vi "Global_MAIN.vi"() -> ()   [LabVIEW 2015]
panel:
  out "tdms file out":refnum<k34>
  in  "Alert email adress":string="jb.fiche@gmail.com" caption="Recipients"
  out "Correct autofocus automatically":bool
  in  "scan step":i32
  out "Stop scan":bool
  out "Stop main vi":bool
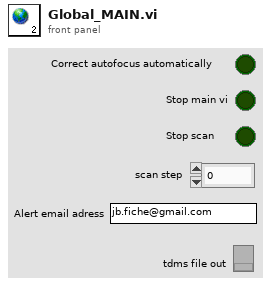
[diagram p1: front panel]
diagram:
